vi "Utility Append Rev to Build Files.vi"(6 "Dash #? (T)":bool, 7 "Executable Name":string, 8 "error in (no error)":errorcluster, 9 "Files Generated by Build in":path[](array[path]), 10 "Top Level/Always Included VIs":path[](array[path]), 11 "Build Specification Name":string) -> (0 "error out":errorcluster, 1 "Files Generated by Build out":path[](array[path]))   [LabVIEW 2015]
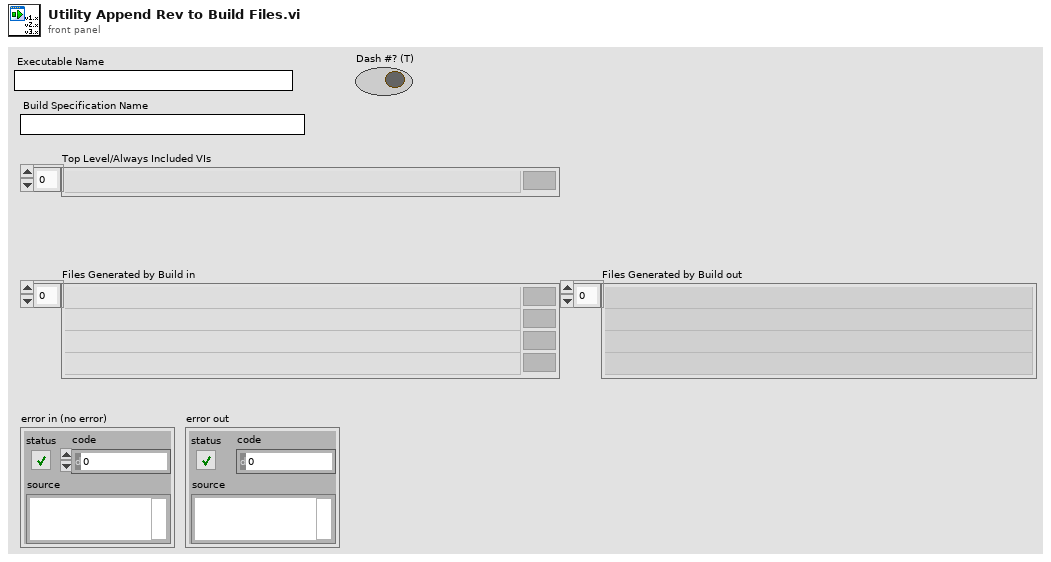
[diagram p1: front panel]
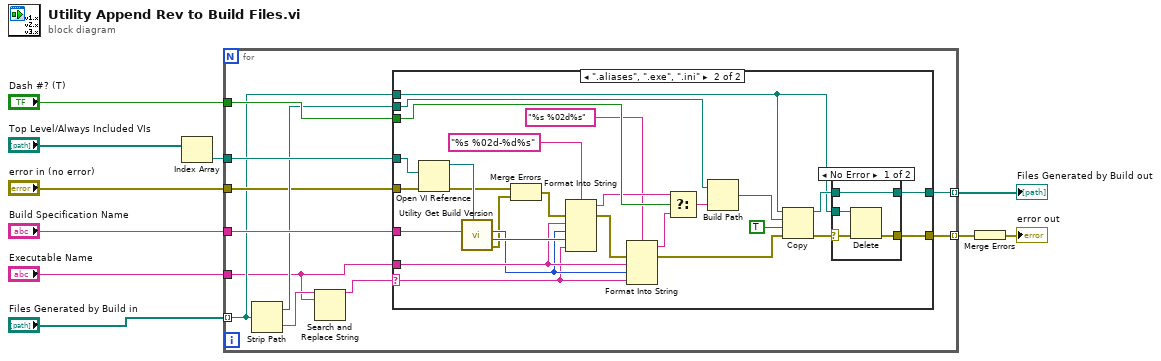
[diagram p0: block diagram]
diagram:
  n1 = Index Array(array="Top Level/Always Included VIs") -> (element=w5:path)  [unwired: 1 in]
  n2 = for {
    tunnel: "Build Specification Name" -> [w21]
    tunnel: "Executable Name" -> [w12]
    tunnel: "Files Generated by Build in" -> [w16] mode=indexing
    tunnel: "Dash #? (T)" -> [w20]
    tunnel: w5 -> [w19]
    tunnel: "error in (no error)" -> [w17]
    tunnel: [w15] -> w3 mode=indexing
    tunnel: [w14] -> w2 mode=indexing
    n3 = Strip Path(path=w16) -> (stripped path=w18:path, name=w13:string)
    n4 = Search and Replace String(input string=w13, search string=w12) -> (result string=w11:string)  [unwired: 6 in, 3 out]
    n5 = case shown="\".aliases\", \".exe\", \".ini\"" w11 {
      selector: w11 -> [_ w41]
      tunnel: w21 -> [_ w50]
      tunnel: w12 -> [_ w43]
      tunnel: w20 -> [_ w46]
      tunnel: w19 -> [_ w39]
      tunnel: w18 -> [_ w38]
      tunnel: w17 -> [w22 w34]
      tunnel: w16 -> [w23 w27]
      tunnel: [w23 w29] -> w15
      tunnel: [w22 w26] -> w14
      frame Default {
      }
      frame ".aliases", ".exe", ".ini" {
        n6 = Open VI Reference(vi path=w39, error in (no error)=w34) -> (vi reference=w49:refnum<vi>, error out=w35:errorcluster)  [unwired: 4 in]
        n7 = call "Utility Get Build Version.vi"("VI Ref in"=w49, "Name of build specification"=w50) -> ("Rev (Build)"=w47:u16, "Version (Fix)"=w42:u16, "error out"=w24:errorcluster)  [unwired: 7 in]
        n8 = Merge Errors(w35, w24) -> (w25:errorcluster)
        n9 = Format Into String(format string="%s %02d-%d%s", error in=w25, w43, w42, w47, w41) -> (resulting string=w45:string, error out=w36:errorcluster)  [unwired: 1 in]
        n10 = Format Into String(format string="%s %02d%s", error in=w36, w43, w42, w41) -> (resulting string=w40:string, error out=w33:errorcluster)  [unwired: 1 in]
        n11 = Select(t=w45, s=w46, f=w40) -> (s? t:f=w37:string)
        n12 = Build Path(base path=w38, name or relative path=w37) -> (appended path=w30:path)
        n13 = Copy(8:w33, 9:TRUE ("overwrite (F)"), 10:w30, 11:w27) -> (0:w32:errorcluster, 3:w28:path)  [unwired: 1 in, 1 out]
        n14 = case shown="No Error" w32 {
          selector: w32 -> [w53 w56]
          tunnel: [w54 w55] -> w29
          tunnel: w28 -> [w54 _]
          tunnel: w27 -> [w52 w55]
          tunnel: [w51 w56] -> w26
          frame No Error {
            n15 = Delete(path (use dialog)=w52, error in=w53) -> (error out=w51:errorcluster)  [unwired: 3 in, 2 out]
          }
          frame Error {
          }
        }
      }
    }
  }
  "Files Generated by Build out" <- w3
  n16 = Merge Errors(w2) -> (→"error out":errorcluster)
